vi "Unpack Auto Array.vi"(0 "Step":i32, 11 "Auton Array":dbl[][](array[numeric])) -> (3 "Action Type":dbl, 4 "Setpoint":dbl, 6 "Time Failsafe":dbl, 8 "Var 1":dbl, 10 "Var 2":dbl, 15 "Var 3":dbl)   [LabVIEW 2016]
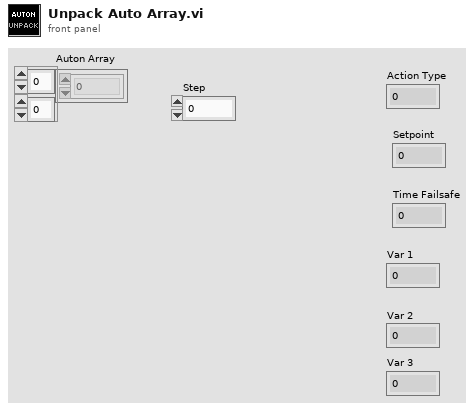
[diagram p1: front panel]
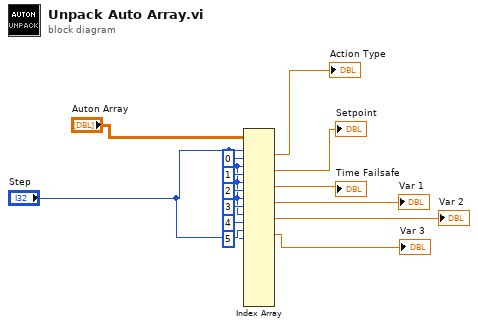
[diagram p0: block diagram]
diagram:
  n1 = Index Array(array="Auton Array", index (row) #1="Step", index (col) #1=0 ("disabled index (col)"), index (row) #2="Step", index (col) #2=1 ("disabled index (col)"), index (row) #3="Step", index (col) #3=2 ("disabled index (col)"), index (row) #4="Step", index (col) #4=3 ("disabled index (col)"), index (row) #5="Step", index (col) #5=4 ("disabled index (col)"), index (row) #6="Step", index (col) #6=5 ("disabled index (col)")) -> (element #1=→"Action Type":dbl, element #2=→"Setpoint":dbl, element #3=→"Time Failsafe":dbl, element #4=→"Var 1":dbl, element #5=→"Var 2":dbl, element #6=→"Var 3":dbl)  [unwired: 8 in, 4 out]
